vi "Destroy TopicFilter.vi"(8 "error in (no error)":errorcluster, 11 "TopicFilter in":refnum<class "TopicFilter.lvclass">) -> (0 "error out":errorcluster, 3 "TopicFilter out":refnum<class "TopicFilter.lvclass">)   [LabVIEW 2013, in "MQTT Server.lvlib" / "TopicFilter.lvclass"]
uses:
  TopicFilter.lvclass
  TopicFilter.lvclass/TopicFilter.ctl
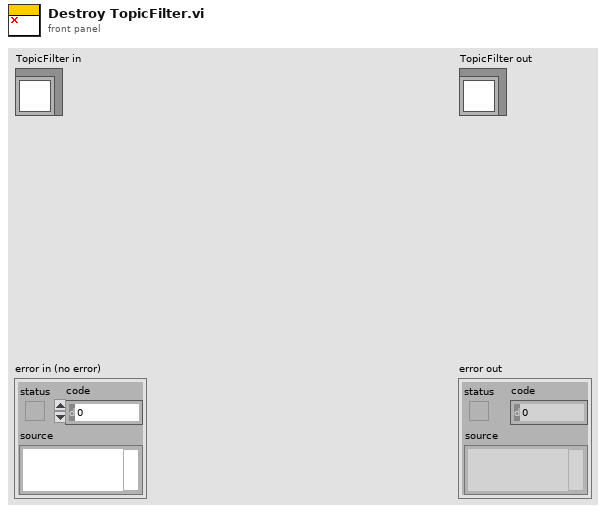
[diagram p1: front panel]
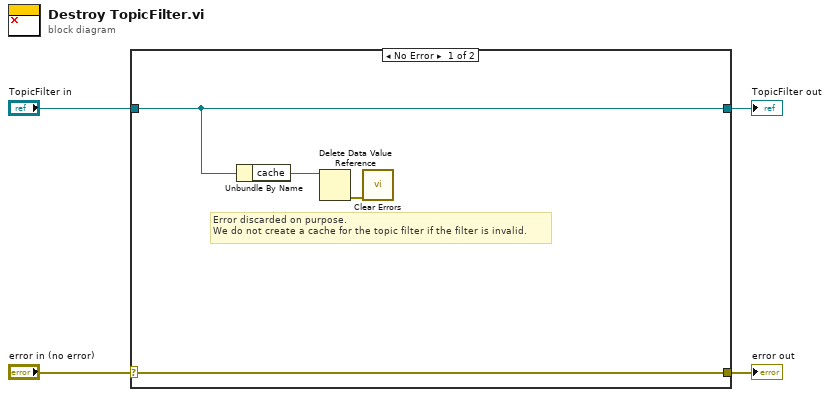
[diagram p0: block diagram]
diagram:
  n1 = case shown="No Error" "error in (no error)" {
    selector: "error in (no error)" -> [w6 w10]
    tunnel: [w6 w10] -> w3
    tunnel: [w8 w9] -> w1
    tunnel: "TopicFilter in" -> [w8 w9]
    frame No Error {
      # "Error discarded on purpose.\nWe do not create a cache for the topic filter if the filter is invalid."
      n2 = Unbundle By Name(w8) -> ("cache"=w7:refnum<data-value>)
      n3 = Delete Data Value Reference(data value reference=w7) -> (error out=w5:errorcluster)  [unwired: 1 in, 1 out]
      n4 = call <vilib>:"Clear Errors.vi"("error in (no error)"=w5) -> ()  [unwired: 6 in, 1 out]
    }
    frame Error {
    }
  }
  "error out" <- w3
  "TopicFilter out" <- w1
